vi "Load-default-configuration.vi"(8 "error in (no error)":errorcluster, 11 "Object ref in":T1) -> (0 "error out":errorcluster, 3 "Object ref out":T1)   [LabVIEW 2013, in "HardwareCharacterization.lvlib" / "HC-Main.lvclass"]
uses:
  HC-Main.lvclass
  Object-reference.ctl
  HC-Main.lvclass/HC-Main.ctl
  Configuration-data.ctl
  Options.ctl
  UI/Control-names.ctl
  Read UI.vi
  Read Status.vi
  Read Base path.vi
  <vilib>/Utility/xml.llb/Read From XML File(string).vi
  UI/Set-control-variant.vi
  UI/HC-UI.lvclass
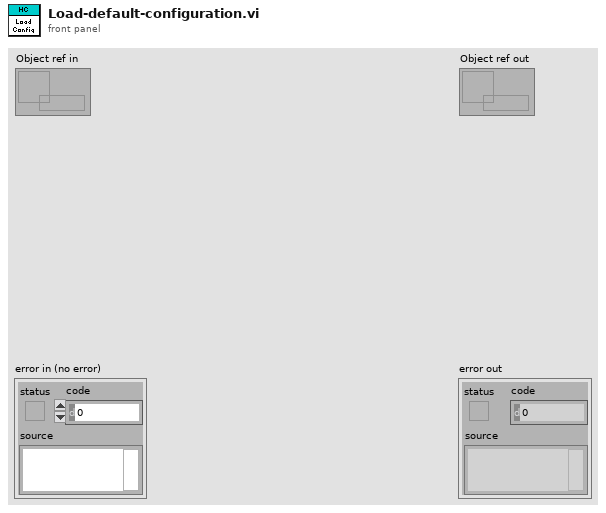
[diagram p1: front panel]
types:
  T1 = typedef "HardwareCharacterization.lvlib/HC-Main.lvclass/Object-reference.ctl" = refnum<data-value>
  T2 = typedef "HardwareCharacterization.lvlib/HC-Main.lvclass/Configuration-data.ctl" = cluster{"Options":T3}
  T3 = typedef "HardwareCharacterization.lvlib/HC-Main.lvclass/Options.ctl" = cluster{"Option 1":bool}
  T4 = typedef "HardwareCharacterization.lvlib/HC-UI.lvclass/Control-names.ctl" = enum16{"Help", "Status", "Load configuration", "Save configuration", "Activate", "Start", "Stop", "Options"}
  T5 = typedef "HardwareCharacterization.lvlib/HC-UI.lvclass/Panes-reference.ctl" = refnum<data-value>
  T6 = typedef "HardwareCharacterization.lvlib/HC-Main.lvclass/Application-status.ctl" = enum16{"Idle", "Initialized", "Configured", "Activated", "Started", "Paused", "Stopped", "Reset", "Error", "Exited"}
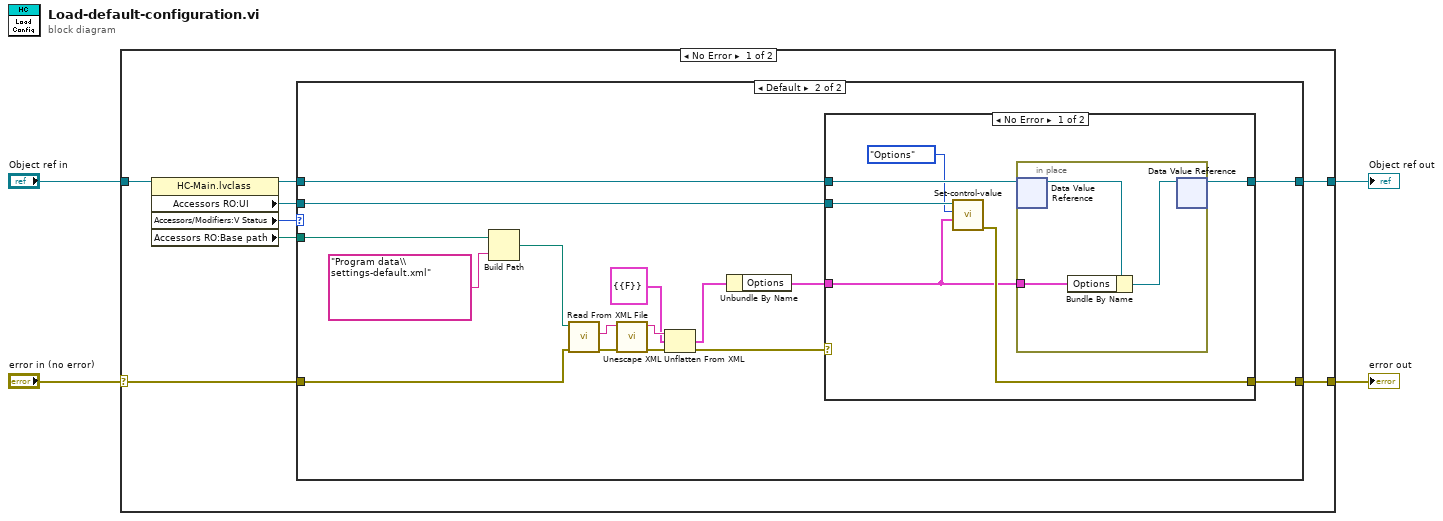
[diagram p0: block diagram]
diagram:
  n1 = case shown="No Error" "error in (no error)" {
    selector: "error in (no error)" -> [w12 w42]
    tunnel: [w8 w42] -> w3
    tunnel: [w7 w41] -> w1
    tunnel: "Object ref in" -> [w11 w41]
    frame No Error {
      n2 = property class="HC-Main.lvclass"(reference=w11) -> (reference out=w9:T1, "Accessors RO:UI"=w10:T5, "Accessors/Modifiers:V Status"=w6:T6, "Accessors RO:Base path"=w5:path)  [unwired: 1 in, 1 out]
      n3 = case shown="Default" w6 {
        tunnel: w12 -> [w14 w18]
        tunnel: w10 -> [_ w16]
        tunnel: w9 -> [w13 w30]
        tunnel: [w14 w29] -> w8
        tunnel: [w13 w23] -> w7
        tunnel: w5 -> [_ w22]
        frame "Activated".."Paused" {
        }
        frame Default {
          n4 = Build Path(base path=w22, name or relative path="Program data\\settings-default.xml") -> (appended path=w19:path)
          n5 = call-poly <vilib>:"Read From XML File.vi"("error in (no error)"=w18, "XML File Path"=w19) -> ("error out"=w28:errorcluster, "XML Elements"=w27:string)  [unwired: 7 in, 1 out]
          n6 = call <vilib>:"Unescape XML.vi"("error in (no error)"=w28, "XML String In"=w27) -> ("error out"=w26:errorcluster, "XML String Out"=w25:string)  [unwired: 8 in]
          n7 = Unflatten From XML(xml string=w25, type=T2 {"Options"={"Option 1"=FALSE}} ("Configuration data"), error in (no error)=w26) -> (value=w21:T2, error out=w15:errorcluster)
          n8 = Unbundle By Name(w21) -> ("Options"=w20:T3)
          n9 = case shown="No Error" w15 {
            tunnel: [w33 _] -> w29
            tunnel: [w36 w40] -> w23
            tunnel: w30 -> [w35 w40]
            tunnel: w20 -> [w31 _]
            tunnel: w16 -> [w34 _]
            frame No Error {
              n10 = call-poly "Set-control-value.vi"("Value"=w31, "Control name"=Control-names."Options", "Panes in"=w34) -> ("error out"=w33:errorcluster)  [unwired: 7 in, 1 out]
              n11 = in-place {
                in-place-border: w31 -> [w37]
                n12 = in-place-dvr #1(w35) -> (w39:refnum<class "HC-Main.lvclass">)  [unwired: 1 out]
                n13 = Bundle By Name(cluster=w39, "Options"=w37) -> (w38:refnum<class "HC-Main.lvclass">)
                n14 = in-place-dvr #1(w38) -> (w36:T1)  [unwired: 1 out]
              }
            }
            frame Error {
            }
          }
        }
      }
    }
    frame Error {
    }
  }
  "error out" <- w3
  "Object ref out" <- w1
